vi "Read Parameters to process.vi"(8 "error in":errorcluster, 11 "State Machine runtime in":refnum<class "State Machine runtime.lvclass">) -> (0 "error out":errorcluster, 2 "Parameters to process":T1, 3 "State Machine runtime out":refnum<class "State Machine runtime.lvclass">)   [LabVIEW 2021, in "State Machine runtime.lvclass"]
uses:
  State Machine runtime.lvclass
  configuration/parameter data indices.ctl
  State Machine runtime.lvclass/State Machine runtime.ctl
  configuration/State Machine configuration.lvclass
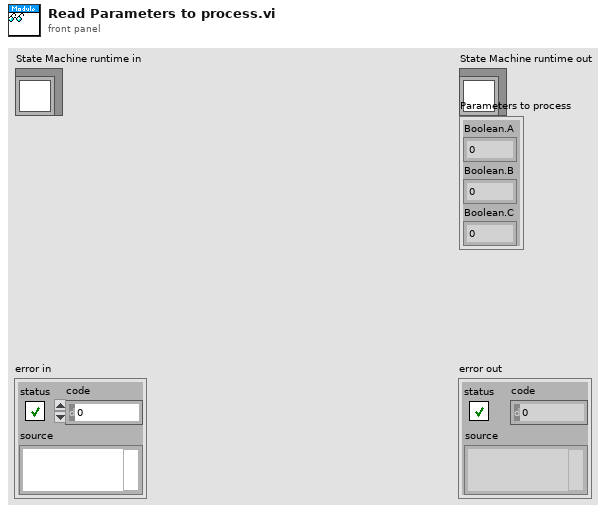
[diagram p1: front panel]
types:
  T1 = typedef "State Machine configuration.lvclass/parameter data indices.ctl" = cluster{"Boolean.A":i32, "Boolean.B":i32, "Boolean.C":i32}
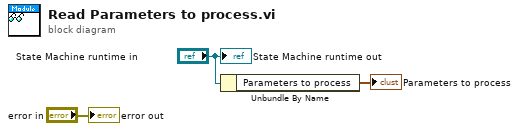
[diagram p0: block diagram]
diagram:
  n1 = Unbundle By Name("State Machine runtime in") -> ("Parameters to process"=→"Parameters to process":T1)
  "error out" <- "error in"
  "State Machine runtime out" <- "State Machine runtime in"
